vi "rd_getX0.vi"(8 "error in (no error)":errorcluster, 10 "absolute time?":bool=TRUE, 11 "WFM":waveform(dbl)) -> (0 "error out":errorcluster, 3 "WFM out":waveform(dbl))   [LabVIEW 2020, in "NI_ExcelFile.lvlib"]
uses:
  <vilib>/express/express shared/NI_ExcelFile/NI_ExcelFile.lvlib
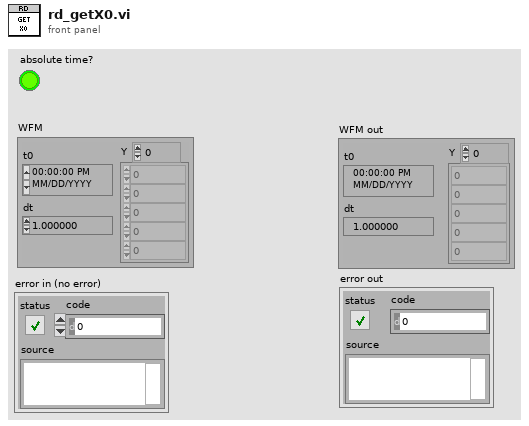
[diagram p1: front panel]
types:
  T1 = typedef "LVDateTimeRec.ctl" = cluster{"fractional second":dbl, "second":i32, "minute":i32, "hour":i32, "day of month":i32, "month":i32, "year":i32, "day of week":i32, "day of year":i32, "DST":i32}
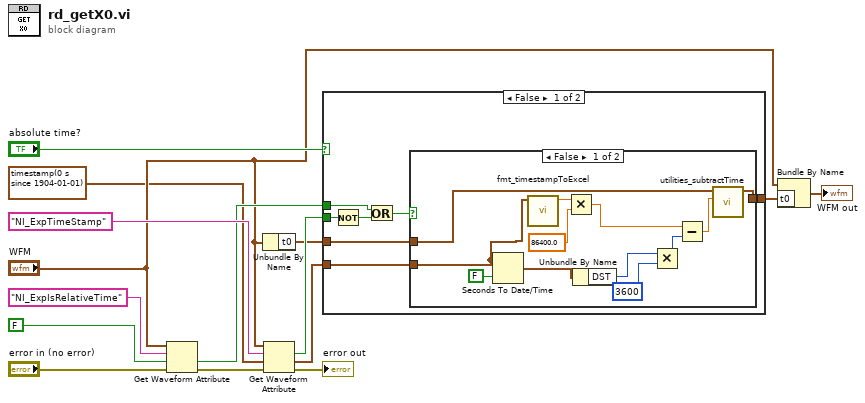
[diagram p0: block diagram]
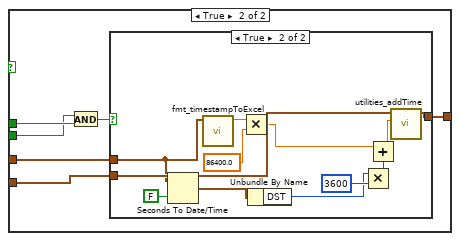
[diagram p3: hidden frame]
diagram:
  n1 = Get Waveform Attribute(4:"error in (no error)", 5:FALSE, 6:"NI_ExpIsRelativeTime" ("name"), 7:"WFM") -> (0:w13:errorcluster, 1:w10:bool)  [unwired: 2 out]
  n2 = Unbundle By Name("WFM") -> ("t0"=w2:timestamp)
  n3 = Get Waveform Attribute(4:w13, 5:timestamp(0 s since 1904-01-01) ("t0"), 6:"NI_ExpTimeStamp" ("name"), 7:"WFM") -> (0:→"error out":errorcluster, 1:w9:timestamp, 2:w5:bool)  [unwired: 1 out]
  n4 = case shown="False" "absolute time?" {
    tunnel: w10 -> [w20 w39]
    tunnel: w9 -> [w22 w41]
    tunnel: [w21 w40] -> w8
    tunnel: w5 -> [w19 w37]
    tunnel: w2 -> [w16 w36]
    frame False {
      n5 = Not(x=w19) -> (.not. x?=w17:bool)
      n6 = Or(x=w20, y=w17) -> (x .or. y?=w18:bool)
      n7 = case shown="False" w18 {
        tunnel: w22 -> [w24 _]
        tunnel: [w25 w35] -> w21
        tunnel: w16 -> [w23 w35]
        frame False {
          n8 = Seconds To Date/Time(time stamp (now)=w24, to UTC (F)=FALSE) -> (date time rec=w31:T1)
          n9 = call <vilib>:"fmt_timestampToExcel.vi"("timestamp"=w24) -> ("Excel timestamp"=w34:dbl)  [unwired: 10 in]
          n10 = Multiply(x=w34, y=86400.0) -> (x*y=w27:dbl)
          n11 = Unbundle By Name(w31) -> ("DST"=w29:i32)
          n12 = Multiply(x=w29, y=3600) -> (x*y=w28:i32)
          n13 = Subtract(x=w27, y=w28) -> (x-y=w26:dbl)
          n14 = call <vilib>:"utilities_subtractTime.vi"("number"=w26, "Time"=w23) -> ("Time out"=w25:timestamp)  [unwired: 9 in]
        }
        frame True {
        }
      }
    }
    frame True {
      n15 = And(x=w37, y=w39) -> (x .and. y?=w38:bool)
      n16 = case shown="True" w38 {
        tunnel: w41 -> [_ w54]
        tunnel: w36 -> [w42 w43]
        tunnel: [w42 w53] -> w40
        frame False {
        }
        frame True {
          n17 = Seconds To Date/Time(time stamp (now)=w43, to UTC (F)=FALSE) -> (date time rec=w49:T1)
          n18 = call <vilib>:"fmt_timestampToExcel.vi"("timestamp"=w43) -> ("Excel timestamp"=w52:dbl)  [unwired: 10 in]
          n19 = Multiply(x=w52, y=86400.0) -> (x*y=w45:dbl)
          n20 = Unbundle By Name(w49) -> ("DST"=w47:i32)
          n21 = Multiply(x=w47, y=3600) -> (x*y=w46:i32)
          n22 = Add(x=w45, y=w46) -> (x+y=w44:dbl)
          n23 = call <vilib>:"utilities_addTime.vi"("number"=w44, "Time"=w54) -> ("Time out"=w53:timestamp)  [unwired: 9 in]
        }
      }
    }
  }
  n24 = Bundle By Name(cluster="WFM", "t0"=w8) -> (→"WFM out":waveform(dbl))
